vi "main.vi"() -> ()   [LabVIEW 2014]
uses:
  <vilib>/MakerHub/LINX/Private/Type Defs/Temperature Units.ctl
  <vilib>/MakerHub/LINX/Public/Peripherals/Digital/Digital Write 1 Chan.vi
  <vilib>/MakerHub/LINX/Public/Peripherals/Digital/Digital Write N Chans.vi
  <vilib>/MakerHub/LINX/Private/Local IO/LinxDigitalWrite.vi
  <vilib>/MakerHub/LINX/Public/Utilities/Check Channel.vi
  <vilib>/MakerHub/LINX/Private/Local IO/Handle Errors.vi
  <vilib>/MakerHub/LINX/Public/Utilities/Open Local.vi
  Global 1.vi
  <vilib>/MakerHub/LINX/Private/Utilties/Generate Error.vi
  <vilib>/MakerHub/LINX/LMH-LINX.lvlib
panel:
  in  "Temp Units":T1
  in  "Paired Resistance":i32
  in  "AI Channel":u8
  in  "Analog Ref Voltage":dbl
  in  "Stop Button":bool
  in  "Digital Output Channel":u8=58
  # "Circuit Schematic"
  # "LINX Device Settings"
  # "Circuit Schematic"
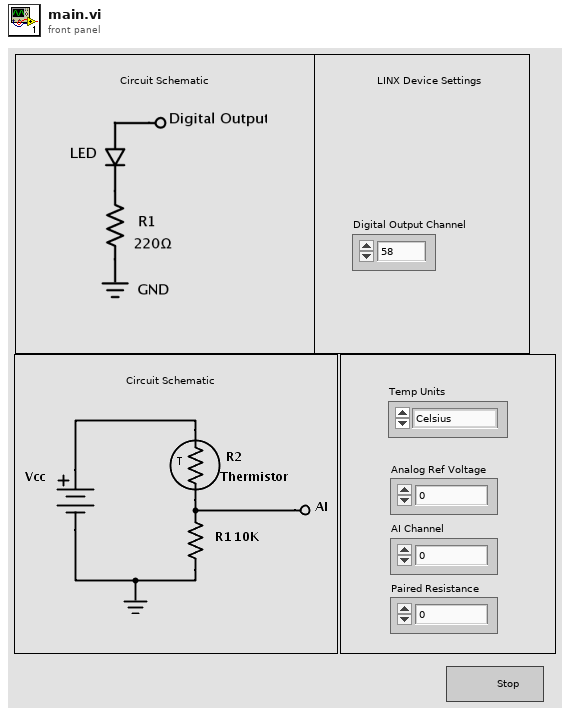
[diagram p1: front panel]
types:
  T1 = typedef "LMH-LINX.lvlib/Temperature Units.ctl" = enum16{"Celsius", "Fahrenheit", "Kelvin", "Rankine"}
  T2 = typedef "LMH-LINX.lvlib/LINX Ref.ctl" = cluster{"IO":T3, "Interface":T4, "LINX Device Config":T5}
  T3 = typedef "LMH-LINX.lvlib/Platform.ctl" = enum16{"Remote", "Local"}
  T4 = typedef "LMH-LINX.lvlib/Interface.ctl" = enum16{"Serial", "TCP"}
  T5 = typedef "LMH-LINX.lvlib/Device.lvlib/LINX Device Config.ctl" = cluster{"Interface":T4, "COM Port":refnum<visa-resource-name>, "TCP Configuration":T6, "Device Family":u8, "Device ID":u8, "Device Name":string, "TCP Ref":refnum<k5>, "Channels":T7}
  T6 = typedef "LMH-LINX.lvlib/Device.lvlib/TCP Config.ctl" = cluster{"IP Address":string, "Port":u16}
  T7 = typedef "LMH-LINX.lvlib/Channels.ctl" = cluster{"DI":u8[], "DO":u8[], "AI":u8[], "AO":u8[], "PWM":u8[], "QE":u8[], "UART":u8[], "I2C 2":u8[], "SPI":u8[], "CAN":u8[], "Servo":u8[], "AI Ref (V)":dbl, "AI Resolution (Bits)":u8, "AO Ref (V)":dbl, "AO Resolution (Bits)":u8}
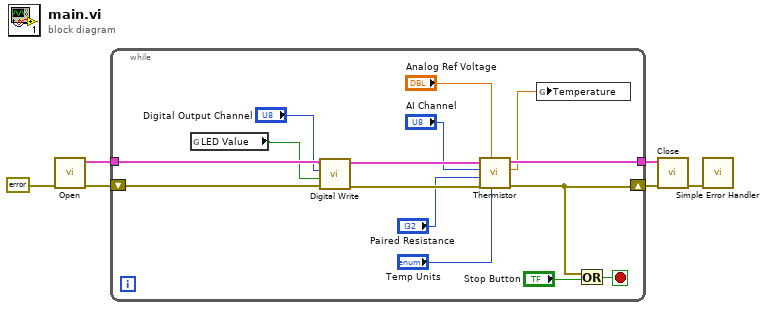
[diagram p0: block diagram]
diagram:
  n1 = call-poly <vilib>:"Open.vi"("Error In"=errorcluster {"status"=FALSE, "code"=0, "source"=""}) -> ("Error Out"=w5:errorcluster, "LINX Resource"=w6:T2)  [unwired: 8 in, 1 out]
  n2 = while {
    tunnel: w6 -> [w19]
    tunnel: [w15] -> w4
    shift-right: [w13] -> w3
    shift-left: w5 -> [w18]
    stop <- w21 stop-if-true
    n3 = global read "Global 1.vi" "LED Value"() -> (w8:bool)
    n4 = call-poly <vilib>:"Digital Write.vi"("Error In"=w18, "Output Value"=w8, "DO Channel"="Digital Output Channel", "LINX Resource"=w19) -> ("Error Out"=w14:errorcluster, "LINX Resource"=w16:T2)  [unwired: 6 in]
    n5 = call <vilib>:"Thermistor.vi"("Units (C)"="Temp Units", "Analog Ref Override"="Analog Ref Voltage", "Error In"=w14, "Paired Resistance"="Paired Resistance", "AI Channel"="AI Channel", "LINX Resource"=w16) -> ("Error Out"=w13:errorcluster, "Temperature"=w7:dbl, "LINX Resource"=w15:T2)  [unwired: 3 in]
    n6 = global write "Global 1.vi" "Temperature"(w7) -> ()
    n7 = Or(x=w13, y="Stop Button") -> (x .or. y?=w21:bool)
  }
  n8 = call <vilib>:"Close.vi"("Error In"=w3, "LINX Resource"=w4) -> ("Error Out"=w2:errorcluster)  [unwired: 9 in]
  n9 = call <vilib>:"Simple Error Handler.vi"("error in (no error)"=w2) -> ()  [unwired: 4 in, 5 out]
